vi "Close Termination.vi"(8 "error in (no error)":errorcluster, 11 "Teststand in":refnum<class "Teststand.lvclass">) -> (0 "error out":errorcluster, 3 "Teststand out":refnum<class "Teststand.lvclass">)   [LabVIEW 2023, in "HardwareAbstractionLayer_LVOOP.lvlib" / "Teststand.lvclass"]
uses:
  Teststand.lvclass
  Teststand.lvclass/Teststand.ctl
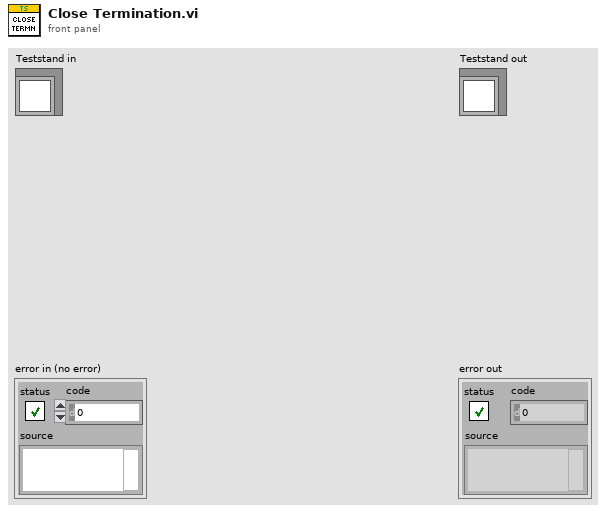
[diagram p1: front panel]
types:
  T1 = typedef "TestStand - Status Monitor.ctl" = cluster{"Sequence Context":refnum<k7>, "Execution":refnum<k7>, "Termination Monitor":refnum<k7>}
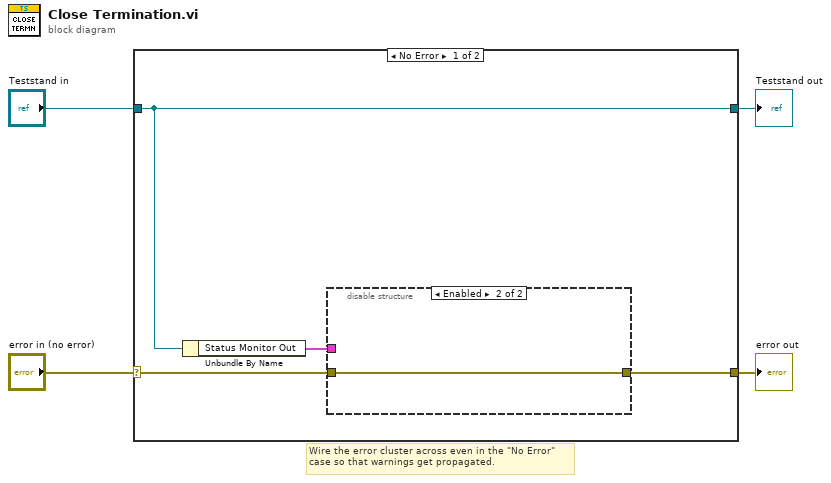
[diagram p0: block diagram]
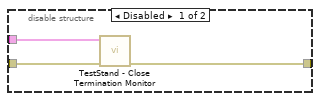
[diagram p2: hidden frame]
diagram:
  # "Wire the error cluster across even in the \"No Error\"\ncase so that warnings get propagated."
  n1 = case shown="No Error" "error in (no error)" {
    selector: "error in (no error)" -> [w8 w14]
    tunnel: [w7 w14] -> w3
    tunnel: [w6 w13] -> w1
    tunnel: "Teststand in" -> [w6 w13]
    frame No Error {
      n2 = Unbundle By Name(w6) -> ("Status Monitor Out"=w5:T1)
      n3 = disable-structure shown="Enabled" {
        disable-tunnel: w8 -> [w11 w12]
        disable-tunnel: [w10 w12] -> w7
        disable-tunnel: w5 -> [w9 _]
        frame Disabled {
          n4 = call <vilib>:"TestStand - Close Termination Monitor.vi"("error in (no error)"=w11, "Status Monitor In"=w9) -> ("error out"=w10:errorcluster)  [unwired: 9 in]
        }
        frame Enabled {
        }
      }
    }
    frame Error {
    }
  }
  "error out" <- w3
  "Teststand out" <- w1
